vi "Move.vi"(8 "error in (no error)":errorcluster, 10 "New Position":cluster{"Row":i8, "Column":i8}, 11 "Amphipod in":refnum<class "Amphipod.lvclass">) -> (0 "error out":errorcluster, 1 "Energy Used":u64, 2 "Old Position":cluster{"Row":i8, "Column":i8}, 3 "Amphipod out":refnum<class "Amphipod.lvclass">)   [LabVIEW 2019, in "23.lvlib" / "Amphipod.lvclass"]
uses:
  Amphipod.lvclass
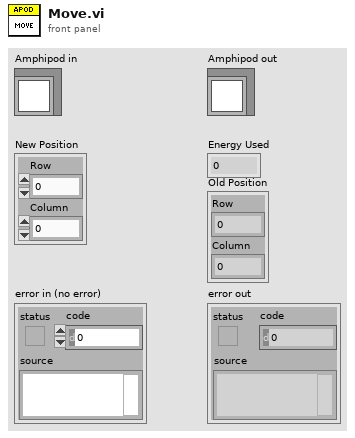
[diagram p1: front panel]
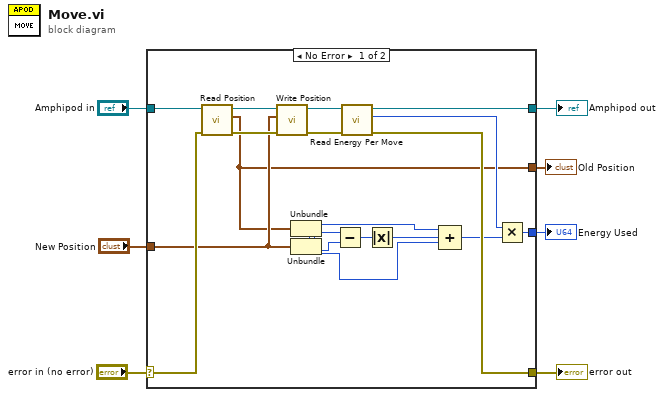
[diagram p0: block diagram]
diagram:
  n1 = case shown="No Error" "error in (no error)" {
    selector: "error in (no error)" -> [w24 w28]
    tunnel: [w22 w28] -> w6
    tunnel: [w26 w27] -> w4
    tunnel: "Amphipod in" -> [w25 w27]
    tunnel: "New Position" -> [w16 _]
    tunnel: [w21 _] -> w2
    tunnel: [w10 _] -> w1
    frame No Error {
      n2 = call-dynamic "Read Position.vi"("error in (no error)"=w24, "Amphipod in"=w25) -> ("error out"=w18:errorcluster, "Position"=w10:cluster{"Row":i8, "Column":i8}, "Amphipod out"=w20:refnum<class "Amphipod.lvclass">)  [unwired: 7 in]
      n3 = call-dynamic "Write Position.vi"("error in (no error)"=w18, "Position"=w16, "Amphipod in"=w20) -> ("error out"=w17:errorcluster, "Amphipod out"=w19:refnum<class "Amphipod.lvclass">)  [unwired: 7 in]
      n4 = Unbundle(w10) -> ("Row"=w15:i8, "Column"=w14:i8)
      n5 = Unbundle(w16) -> ("Row"=w8:i8, "Column"=w9:i8)
      n6 = Subtract(x=w14, y=w9) -> (x-y=w13:i8)
      n7 = call-dynamic "Read Energy Per Move.vi"("error in (no error)"=w17, "Amphipod in"=w19) -> ("error out"=w22:errorcluster, "Energy Per Move"=w23:u16, "Amphipod out"=w26:refnum<class "Amphipod.lvclass">)  [unwired: 7 in]
      n8 = Absolute Value(x=w13) -> (abs(x)=w12:i8)
      n9 = Compound Arithmetic op=ADD(w15, w12, w8) -> (w11:i8)
      n10 = Multiply(x=w23, y=w11) -> (x*y=w21:u16)
    }
    frame Error {
    }
  }
  "error out" <- w6
  "Amphipod out" <- w4
  "Energy Used" <- w2
  "Old Position" <- w1
